vi "Start Instances.vi"(7 "Information":refnum<vi>, 8 "error in (no error)":errorcluster, 9 "interval(50ms)":u32=50) -> (0 "error out":errorcluster)   [LabVIEW 2020, in "CSM-ModuleManager.lvlib"]
uses:
  CSM-ModuleManager.lvlib
  Operation.ctl
  <userlib>/_NEVSTOP/Communicable State Machine(CSM)/addons/INI-Static-Variable-Support/INI-Static-Variable-Support.lvlib
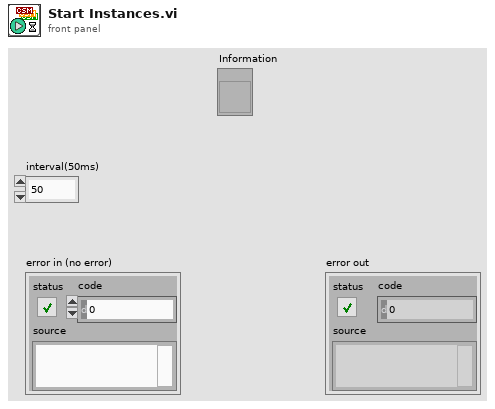
[diagram p1: front panel]
types:
  T1 = typedef "CSM-ModuleManager.lvlib/Operation.ctl" = enum16{"Register", "UnRegister", "Load Config", "Get"}
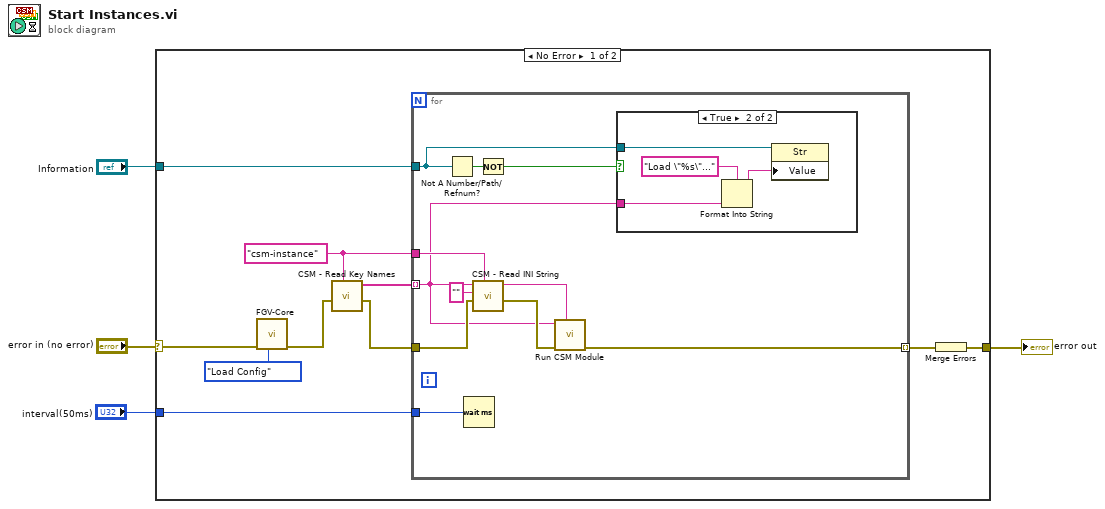
[diagram p0: block diagram]
diagram:
  n1 = case shown="No Error" "error in (no error)" {
    selector: "error in (no error)" -> [w7 w30]
    tunnel: [w14 w30] -> w4
    tunnel: "Information" -> [w9 _]
    tunnel: "interval(50ms)" -> [w8 _]
    frame No Error {
      w11 = "csm-instance" ("Section Name (\"\" as Default)")
      n2 = call "FGV-Core.vi"("Enum"=Operation."Load Config", "error in (no error)"=w7) -> ("error out"=w6:errorcluster)  [unwired: 7 in, 2 out]
      n3 = call <userlib>:"CSM - Read Key Names.vi"("Section Name (\"\" as Default)"=w11, "error in (no error)"=w6) -> ("error out"=w10:errorcluster, "Keys"=w12:string[])  [unwired: 6 in]
      n4 = for {
        tunnel: w11 -> [w24]
        tunnel: w12 -> [w15] mode=indexing
        tunnel: w10 -> [w25]
        tunnel: [w21] -> w13 mode=indexing
        tunnel: w9 -> [w18]
        tunnel: w8 -> [w16]
        n5 = Not A Number/Path/Refnum?(number/path/refnum=w18) -> (NaN/Path/Refnum?=w20:bool)
        n6 = Wait (ms)(milliseconds to wait=w16) -> ()  [unwired: 1 out]
        n7 = call <userlib>:"CSM - Read INI String.vi"("Section Name (\"\" as Default)"=w24, "error in (no error)"=w25, "Default Value"="", "Variable Name"=w15) -> ("error out"=w22:errorcluster, "Value"=w17:string)  [unwired: 3 in, 1 out]
        n8 = Not(x=w20) -> (.not. x?=w19:bool)
        n9 = call "Run CSM Module.vi"("CSM-Module"=w17, "Error in"=w22, "CSM-Instance"=w15) -> ("Error out"=w21:errorcluster)  [unwired: 8 in]
        n10 = case shown="True" w19 {
          tunnel: w18 -> [_ w29]
          tunnel: w15 -> [_ w27]
          frame False {
          }
          frame True {
            n11 = Format Into String(format string="Load \"%s\"...", w27) -> (resulting string=w26:string)  [unwired: 2 in, 1 out]
            n12 = property class="Str"(reference=w29, "Value"=w26) -> ()  [unwired: 1 in, 2 out]
          }
        }
      }
      n13 = Merge Errors(w13) -> (w14:errorcluster)
    }
    frame Error {
    }
  }
  "error out" <- w4
